vi "JumpToAnotherVI.vi"(8 "错误输入（无错误）":errorcluster, 11 "VI名称":string="Main.vi") -> (0 "错误输出":errorcluster)   [LabVIEW 2014]
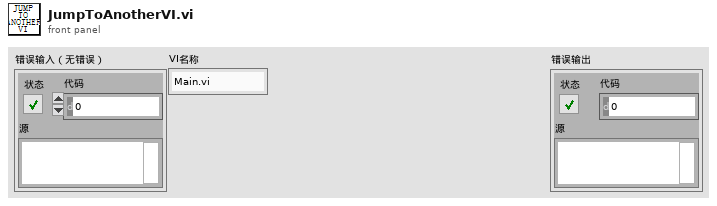
[diagram p1: front panel]
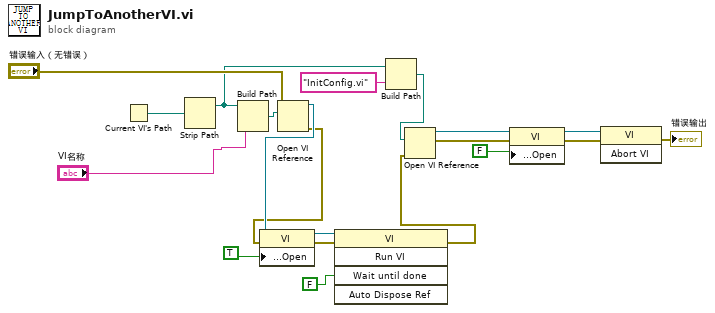
[diagram p0: block diagram]
diagram:
  n1 = Current VI's Path() -> (path=w7:path)
  n2 = Strip Path(path=w7) -> (stripped path=w6:path)  [unwired: 1 out]
  n3 = Build Path(base path=w6, name or relative path="VI名称") -> (appended path=w20:path)
  n4 = Open VI Reference(vi path=w20, error in (no error)="错误输入（无错误）") -> (vi reference=w15:refnum<vi>, error out=w14:errorcluster)  [unwired: 4 in]
  n5 = property on="Property Node" class="VI"(reference=w15, error in=w14, "Front Panel Window:Open"=TRUE) -> (reference out=w18:refnum<vi>, error out=w17:errorcluster)
  n6 = invoke class="VI" method="Run VI"(reference=w18, error in=w17, "Wait until done"=FALSE) -> (error out=w10:errorcluster)  [unwired: 2 in, 4 out]
  n7 = Build Path(base path=w6, name or relative path="InitConfig.vi" ("名称或相对路径")) -> (appended path=w4:path)
  n8 = Open VI Reference(vi path=w4, error in (no error)=w10) -> (vi reference=w13:refnum<vi>, error out=w11:errorcluster)  [unwired: 4 in]
  n9 = property on="Property Node" class="VI"(reference=w13, error in=w11, "Front Panel Window:Open"=FALSE) -> (reference out=w3:refnum<vi>, error out=w2:errorcluster)
  n10 = invoke class="VI" method="Abort VI"(reference=w3, error in=w2) -> (error out=→"错误输出":errorcluster)  [unwired: 1 in, 2 out]
